vi "Actor Core.vi"(8 "error in":errorcluster, 11 "Evaporative Cooler":refnum<class "Evaporative Cooler.lvclass">) -> (0 "error out":errorcluster, 3 "Actor out":refnum<class "Actor.lvclass">)   [LabVIEW 2018, in "Evaporative Cooler.lvlib" / "Evaporative Cooler.lvclass"]
doc: "This is Actor Core.vi, the main message handling loop for Actors. An actor usually just sits in this loop and processes messages as they arrive. Any error returned by the message Do.vi call will stop the loop, with error code 43 as the canonical signal to stop with no error sent to caller. Descendants may override that in Handle Error.vi."
uses:
  Evaporative Cooler.lvclass
  C:/Program Files (x86)/National Instruments/LabVIEW 2018/vi.lib/ActorFramework/Actor/Actor.lvclass
  C:/GitClones/LGP5-Resources/Frameworks/Actor Framework/Feedback Evaporative Cooler/Timed Loop Actor/Timed Loop Actor/Timed Loop Actor.lvclass
  <vilib>/ActorFramework/Actor/Actor.lvclass
  Cooler Update Fan Status Msg/Cooler Update Fan Status Msg.lvclass
  C:/GitClones/LGP5-Resources/Frameworks/Actor Framework/Feedback Evaporative Cooler/Dual Fan/Update Fan Status Msg/Update Fan Status Msg.lvclass
  Cooler Update Water Level Msg/Cooler Update Water Level Msg.lvclass
  C:/GitClones/LGP5-Resources/Frameworks/Actor Framework/Feedback Evaporative Cooler/Water Level/Update Water Level Msg/Update Water Level Msg.lvclass
  Timed Loop Actor/Timed Loop Actor/Timed Loop Actor.lvclass/Timed Loop Actor.ctl
  Dual Fan/Dual Fan/Dual Fan.lvclass/Dual Fan.ctl
  Water Level/Water Level.lvclass/Water Level.ctl
  Evaporative Cooler.lvclass/Evaporative Cooler.ctl
  Dual Fan/Dual Fan/Dual Fan.lvclass
  Water Level/Water Level.lvclass
  C:/GitClones/LGP5-Resources/Frameworks/Actor Framework/Feedback Evaporative Cooler/Level Controller/Level Controller/Level Controller.lvclass
  <vilib>/Utility/LVClass/Get LV Class Path.vi
  Cooler/Cooler/Cooler.lvclass
  Level Controller/Level Controller/Level Controller.lvclass
  Timed Loop Actor/Timed Loop Actor/Timed Loop Actor.lvclass
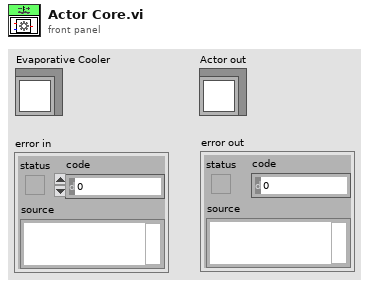
[diagram p1: front panel]
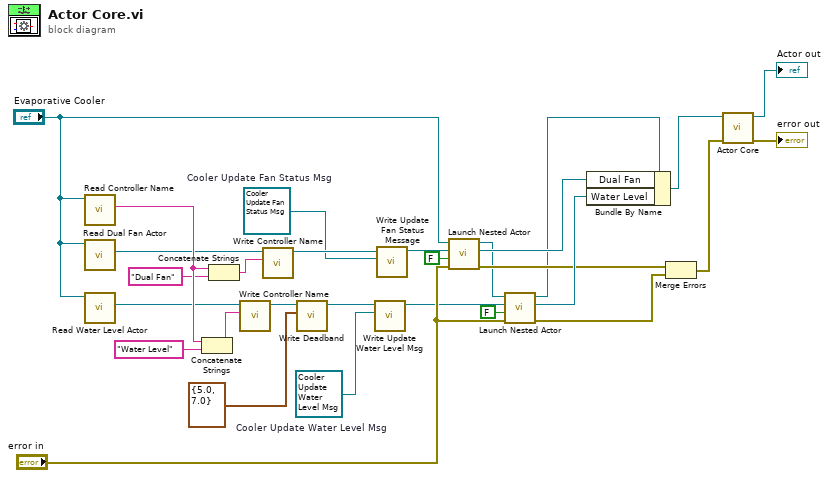
[diagram p0: block diagram]
diagram:
  w9 = refnum<class "Cooler Update Water Level Msg.lvclass"> refnum  # Cooler Update Water Level Msg
  w14 = refnum<class "Cooler Update Fan Status Msg.lvclass"> refnum  # Cooler Update Fan Status Msg
  n1 = call "Read Controller Name.vi"("Timed Loop Controller"="Evaporative Cooler") -> ("Controller Name"=w18:string)  [unwired: 10 in]
  n2 = call-dynamic "Read Dual Fan Actor.vi"("Evaporative Cooler"="Evaporative Cooler") -> ("Dual Fan"=w13:refnum<class "Dual Fan.lvclass">)  [unwired: 10 in]
  n3 = call-dynamic "Read Water Level Actor.vi"("Evaporative Cooler"="Evaporative Cooler") -> ("Water Level"=w12:refnum<class "Water Level.lvclass">)  [unwired: 10 in]
  n4 = Concatenate Strings(w18, "Water Level" ("string")) -> (w19:string)
  n5 = Concatenate Strings(w18, "Dual Fan" ("string")) -> (w15:string)
  n6 = call "Write Controller Name.vi"("Controller Name"=w19, "Timed Loop Controller in"=w12) -> ("Timed Loop Controller out"=w11:refnum<class "Water Level.lvclass">)  [unwired: 9 in]
  n7 = call "Write Controller Name.vi"("Controller Name"=w15, "Timed Loop Controller in"=w13) -> ("Timed Loop Controller out"=w20:refnum<class "Dual Fan.lvclass">)  [unwired: 9 in]
  n8 = call "Write Deadband.vi"("Deadband"=cluster{"LO":dbl, "HI":dbl} {"LO"=5.0, "HI"=7.0}, "Level Controller in"=w11) -> ("Level Controller out"=w10:refnum<class "Water Level.lvclass">)  [unwired: 8 in, 1 out]
  n9 = call "Write Update Water Level Msg.vi"("Update Water Level Msg"=w9, "Water Level in"=w10) -> ("Water Level out"=w6:refnum<class "Water Level.lvclass">)  [unwired: 9 in]
  n10 = call "Write Update Fan Status Message.vi"("Update Msg"=w14, "Dual Fan in"=w20) -> ("Dual Fan out"=w7:refnum<class "Dual Fan.lvclass">)  [unwired: 9 in]
  n11 = call <vilib>:"Launch Nested Actor.vi"("error in (no error)"="error in", "Auto-stop? (T)"=FALSE, "Nested Actor"=w7, "Caller Actor in"="Evaporative Cooler") -> ("error out"=w24:errorcluster, "Nested Actor's Enqueuer"=w26:refnum<class "Message Enqueuer.lvclass">, "Caller Actor out"=w5:refnum<class "Evaporative Cooler.lvclass">)  [unwired: 5 in]
  n12 = call <vilib>:"Launch Nested Actor.vi"("error in (no error)"="error in", "Auto-stop? (T)"=FALSE, "Nested Actor"=w6, "Caller Actor in"=w5) -> ("error out"=w23:errorcluster, "Nested Actor's Enqueuer"=w27:refnum<class "Message Enqueuer.lvclass">, "Caller Actor out"=w3:refnum<class "Evaporative Cooler.lvclass">)  [unwired: 5 in]
  n13 = Bundle By Name(cluster=w3, "Dual Fan"=w26, "Water Level"=w27) -> (w25:refnum<class "Evaporative Cooler.lvclass">)
  n14 = Merge Errors(w24, w23) -> (w22:errorcluster)
  n15 = call-parent "Actor Core.vi"("error in"=w22, "Timed Loop Controller"=w25) -> ("error out"=→"error out":errorcluster, "Actor out"=→"Actor out":refnum<class "Actor.lvclass">)  [unwired: 8 in]
